vi "Day 7.2 - .vi"(11 "input":string[](array[string])) -> (3 "output":u64)   [LabVIEW 2021]
uses:
  5c7be67d-aeaf-4465-b345-c2cb8e4da54c.vi
  <vilib>/Comparison/Less/Less Functor/Less Functor.lvclass
panel:
  out "Space to be found":i32
  out "Unused space":i32
  out "Space used":i32
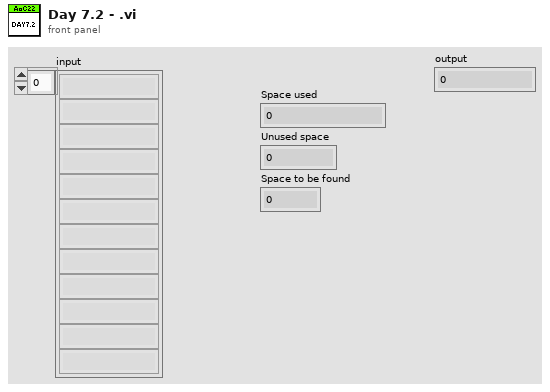
[diagram p1: front panel]
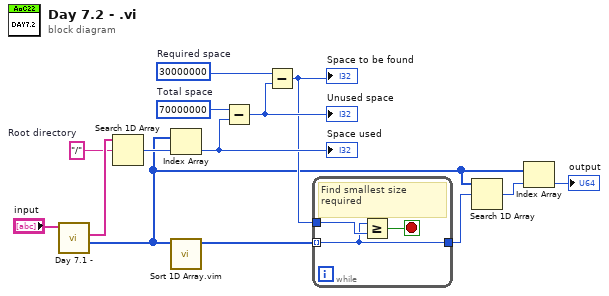
[diagram p0: block diagram]
diagram:
  w12 = "/"  # Root directory
  w8 = 30000000  # Required space
  w10 = 70000000  # Total space
  n1 = call "Day 7.1 - .vi"("input"="input") -> ("Sizes"=w1:i32[], "Dirs"=w13:string[])  [unwired: 8 in, 1 out]
  n2 = Search 1D Array(1D array=w13, element=w12) -> (index of element=w11:i32)  [unwired: 1 in]
  n3 = Index Array(array=w1, index=w11) -> (element=w9:i32)
  "Space used" <- w9
  n4 = call "Sort 1D Array.vim"("unsorted array"=w1) -> ("sorted array"=w6:i32[])  [unwired: 10 in]
  n5 = Subtract(x=w10, y=w9) -> (x-y=w7:i32)
  "Unused space" <- w7
  n6 = Subtract(x=w8, y=w7) -> (x-y=w5:i32)
  "Space to be found" <- w5
  n7 = while {
    tunnel: w6 -> [w15] mode=indexing
    tunnel: w5 -> [w17]
    tunnel: [w15] -> w4
    stop <- w16 stop-if-true
    # "Find smallest size required"
    n8 = Greater Or Equal?(x=w15, y=w17) -> (x >= y?=w16:bool)
  }
  n9 = Search 1D Array(1D array=w1, element=w4) -> (index of element=w3:i32)  [unwired: 1 in]
  n10 = Index Array(array=w1, index=w3) -> (element=→"output":i32)
